vi "Delete Element.vi"(8 "error in (no error)":errorcluster, 9 "Variant":variant, 10 "Key":string, 11 "SMO.Dictionary in":refnum<class "SMO.Dictionary.lvclass">) -> (0 "error out":errorcluster, 1 "Deleted Element":T1, 3 "SMO.Dictionary out":refnum<class "SMO.Dictionary.lvclass">)   [LabVIEW 2013, in "SMO.Dictionary.lvlib" / "SMO.Dictionary.lvclass"]
uses:
  SMO.Dictionary.lvclass
  Typedefs/PrivateEvents--SMO.Dictionary.KeyValue-Pair.ctl
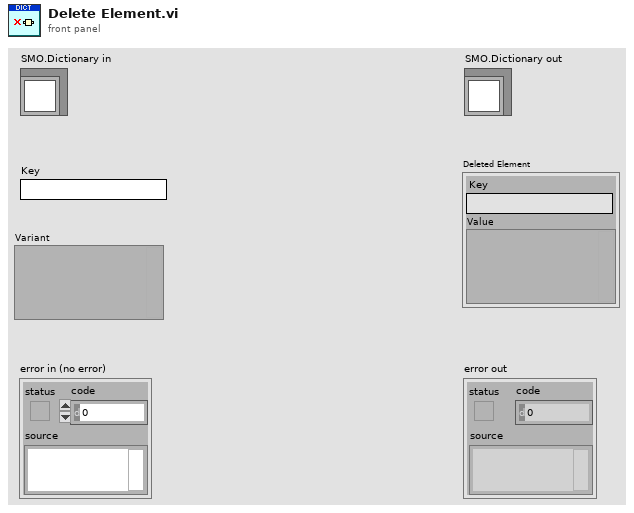
[diagram p1: front panel]
types:
  T1 = typedef "SMO.Dictionary.lvlib/SMO.Dictionary.lvclass/PrivateEvents--SMO.Dictionary.KeyValue-Pair.ctl" = cluster{"Key":string, "Value":variant}
  T2 = typedef "SMO.Dictionary.lvlib/SMO.Dictionary.lvclass/PublicEvents--Cluster.ctl" = cluster{"Cleared":refnum<user-event>, "Deleted":refnum<user-event>, "Updated":refnum<user-event>}
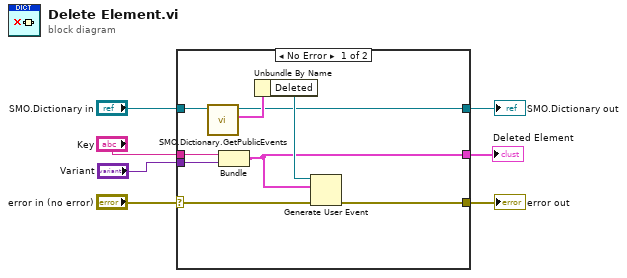
[diagram p0: block diagram]
diagram:
  n1 = case shown="No Error" "error in (no error)" {
    selector: "error in (no error)" -> [w13 w18]
    tunnel: [w12 w18] -> w6
    tunnel: [w14 w17] -> w7
    tunnel: "SMO.Dictionary in" -> [w9 w17]
    tunnel: "Key" -> [w11 _]
    tunnel: "Variant" -> [w10 _]
    tunnel: [w8 _] -> w1
    frame No Error {
      n2 = call "SMO.Dictionary.GetPublicEvents.vi"("SMO.Dictionary in"=w9) -> ("Public Events"=w16:T2, "SMO.Dictionary out"=w14:refnum<class "SMO.Dictionary.lvclass">)  [unwired: 8 in, 1 out]
      n3 = Bundle("Key"=w11, "Variant"=w10) -> (w8:cluster{"Key":string, "Variant":variant})  [unwired: 1 in]
      n4 = Unbundle By Name(w16) -> ("Deleted"=w15:refnum<user-event>)
      n5 = Generate User Event(user event=w15, event data cluster=w8, error in=w13) -> (error out=w12:errorcluster)  [unwired: 1 in, 1 out]
    }
    frame Error {
    }
  }
  "error out" <- w6
  "SMO.Dictionary out" <- w7
  "Deleted Element" <- w1
